vi "Repeat Key.vi"(8 "error in (no error)":errorcluster, 10 "Key-Value Pair":T1, 11 "Parameter to Hardware Map in":refnum<class "Parameter to Hardware Map.lvclass">) -> (0 "error out":errorcluster, 2 "Repeat?":bool, 3 "Parameter to Hardware Map out":refnum<class "Parameter to Hardware Map.lvclass">)   [LabVIEW 2020, in "Parameter to Hardware Map.lvclass"]
doc: "Checks if the given key is a repeat of one in the map"
uses:
  Parameter to Hardware Map.lvclass
  Controller/Generic Plugin.lvclass
  Pair.ctl
panel:
  out "Numeric":i32
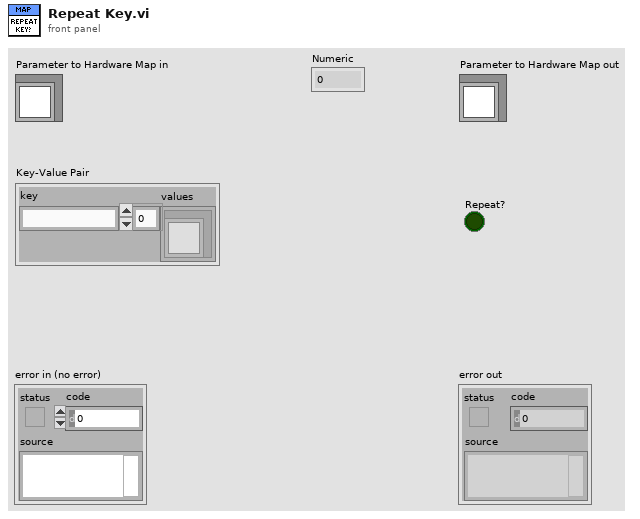
[diagram p1: front panel]
types:
  T1 = typedef "Parameter to Hardware Map.lvclass/Pair.ctl" = cluster{"key":string, "values":refnum<class "Generic Plugin.lvclass">[]}
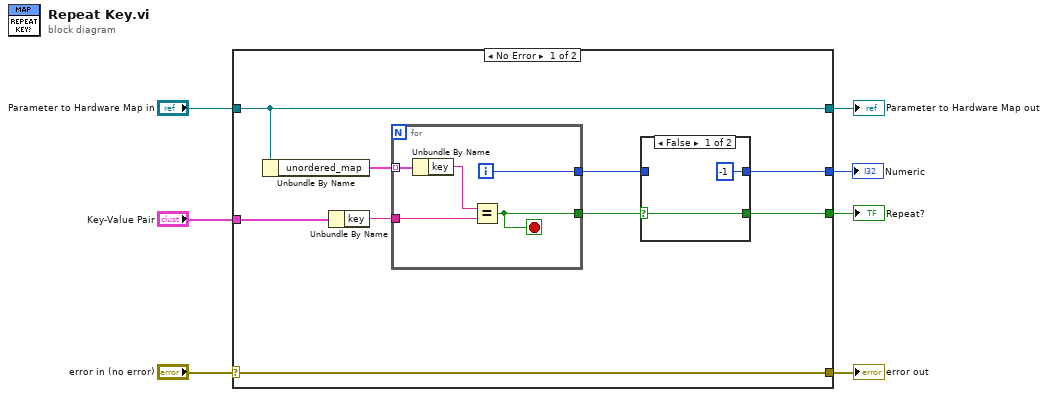
[diagram p0: block diagram]
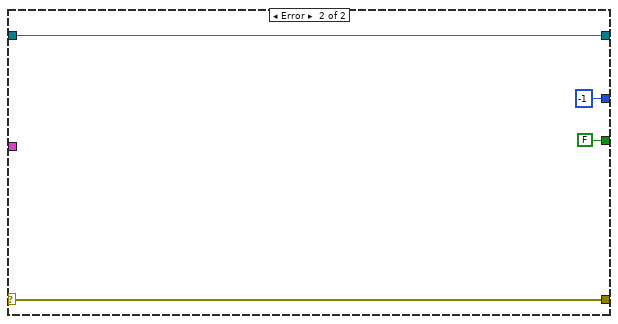
[diagram p3: hidden frame]
diagram:
  n1 = case shown="No Error" "error in (no error)" {
    selector: "error in (no error)" -> [w16 w29]
    tunnel: [w16 w29] -> w6
    tunnel: [w14 w28] -> w4
    tunnel: "Parameter to Hardware Map in" -> [w14 w28]
    tunnel: "Key-Value Pair" -> [w15 _]
    tunnel: [w10 FALSE] -> w2
    tunnel: [w8 -1] -> w1
    frame No Error {
      n2 = Unbundle By Name(w14) -> ("unordered_map"=w13:T1[])
      n3 = Unbundle By Name(w15) -> ("key"=w12:string)
      n4 = for {
        tunnel: w13 -> [w25] mode=indexing
        tunnel: w12 -> [w23]
        tunnel: [w22] -> w11
        tunnel: [w21] -> w9
        i -> [w21]
        stop <- w22 stop-if-true
        n5 = Unbundle By Name(w25) -> ("key"=w24:string)
        n6 = Equal?(x=w24, y=w23) -> (x = y?=w22:bool)
      }
      n7 = case shown="False" w11 {
        selector: w11 -> [w17 w20]
        tunnel: [w17 w20] -> w10
        tunnel: w9 -> [_ w19]
        tunnel: [-1 w19] -> w8
        frame False {
        }
        frame True {
        }
      }
    }
    frame Error {
    }
  }
  "error out" <- w6
  "Parameter to Hardware Map out" <- w4
  "Repeat?" <- w2
  "Numeric" <- w1
